vi "TurnOn_PowerSupply.vi"(5 "Channel_B":T1, 7 "Channel_A":T1, 8 "error in (no error)":errorcluster {"code" format="%.0x"}, 10 "Keysight PS":bool, 11 "VISA resource name":refnum<visa-resource-name>) -> (0 "error out":errorcluster {"code" format="%.0x"}, 3 "VISA resource name out":refnum<visa-resource-name>)   [LabVIEW 2018]
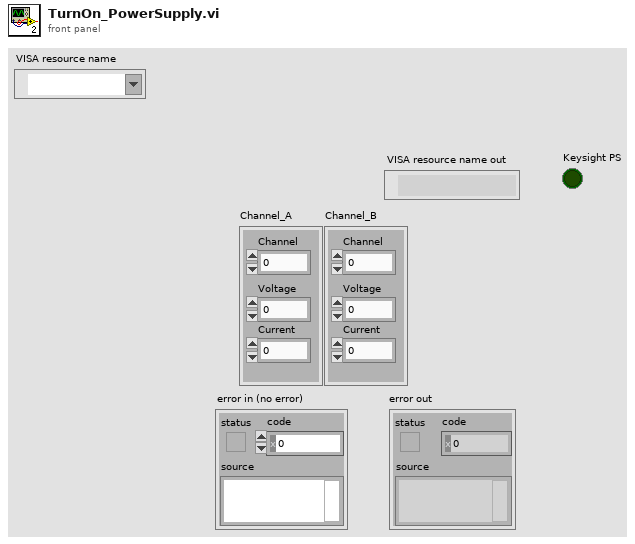
[diagram p1: front panel]
types:
  T1 = cluster{"Channel":dbl, "Voltage":dbl, "Current":dbl}
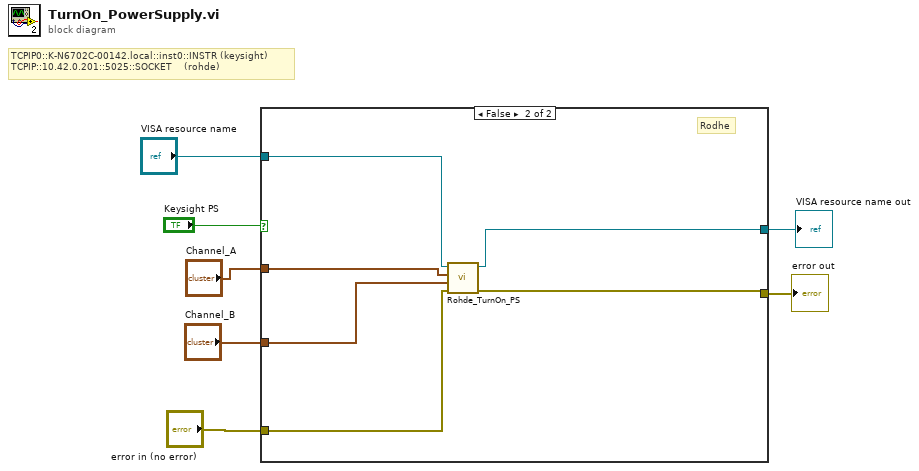
[diagram p0: block diagram]
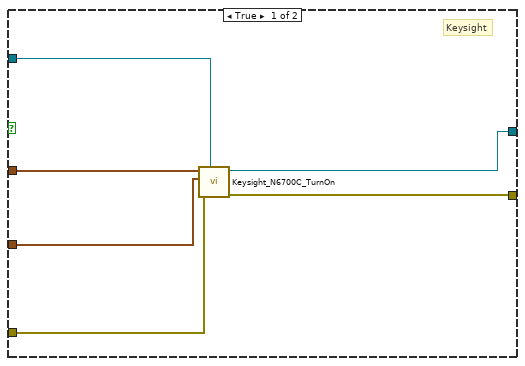
[diagram p2: hidden frame]
diagram:
  # "TCPIP0::K-N6702C-00142.local::inst0::INSTR (keysight)\nTCPIP::10.42.0.201::5025::SOCKET    (rohde)"
  n1 = case shown="False" "Keysight PS" {
    tunnel: "error in (no error)" -> [w13 w17]
    tunnel: [w12 w18] -> w6
    tunnel: [w11 w19] -> w5
    tunnel: "Channel_A" -> [w10 w16]
    tunnel: "Channel_B" -> [w9 w15]
    tunnel: "VISA resource name" -> [w8 w14]
    frame True {
      # "Keysight"
      n2 = call "Keysight_N6700C_TurnOn.vi"("error in (no error)"=w13, "VISA resource name"=w8, "Channel_B"=w9, "Channel_A"=w10) -> ("error out"=w12:errorcluster, "VISA resource name out"=w11:refnum<visa-resource-name>)  [unwired: 6 in]
    }
    frame False {
      # "Rodhe"
      n3 = call "Rohde_TurnOn_PS.vi"("error in (no error)"=w17, "Channel_B"=w15, "Channel_A"=w16, "VISA resource name"=w14) -> ("error out"=w18:errorcluster, "VISA resource name out"=w19:refnum<visa-resource-name>)  [unwired: 6 in]
    }
  }
  "error out" <- w6
  "VISA resource name out" <- w5
